vi "BMark_Highlight Object.vi"(6 "Poly Path":path, 7 "Analysis App Ref":refnum<vi>, 8 "error in (no error)":errorcluster, 10 "Run Prog?":bool, 11 "GObj Refnum":refnum<vi>) -> (0 "error out":errorcluster)   [LabVIEW 2016]
uses:
  <resource>/dialog/BookmarkManager/managers/Default/globals/BMark_User Visible Strings.vi
panel:
  # "Copied from VIAnRes Highlight Object.vi"
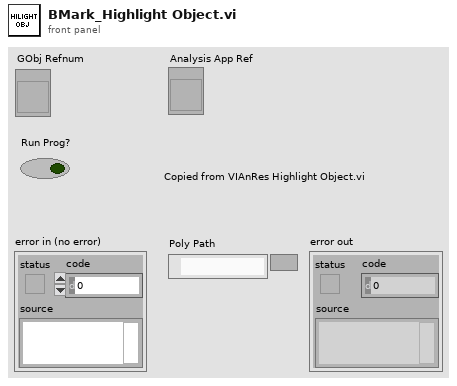
[diagram p1: front panel]
types:
  T1 = enum32{"invalid VI type", "Standard VI", "Control VI", "Global VI", "Polymorphic VI", "Configuration VI"}
  T2 = enum32{"Bad", "Idle", "Run top level", "Running"}
  T3 = enum32{"invalid VI type", "Standard VI", "Control VI", "Global VI", "Polymorphic VI", "Configuration VI", "SubSystem", "Facade VI", "Method VI", "Statechart Diagram VI"}
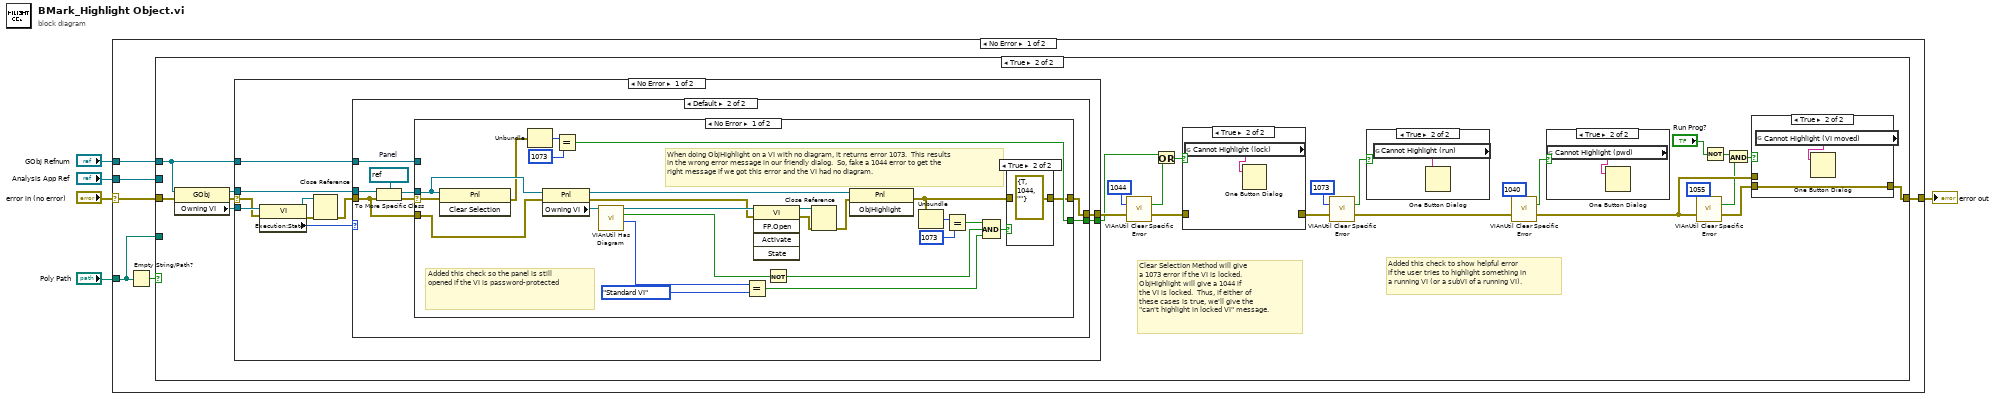
[diagram p0: block diagram]
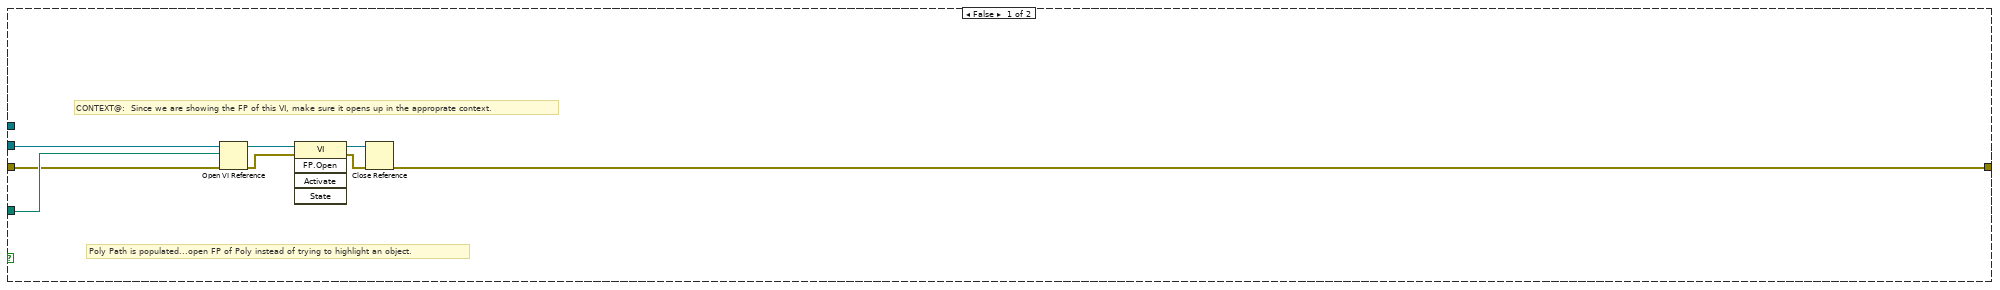
[diagram p2: hidden frame]
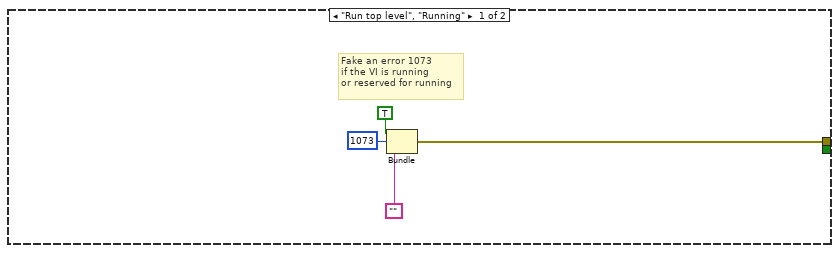
[diagram p3: hidden frame]
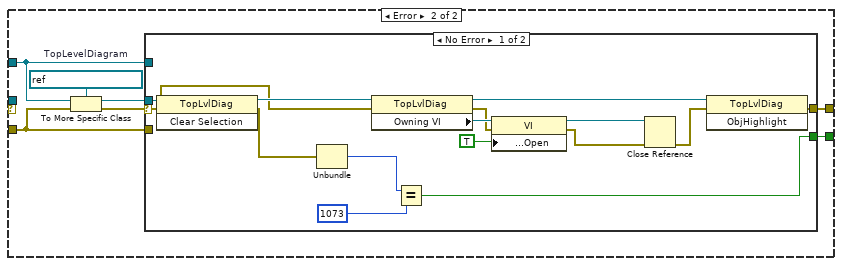
[diagram p5: hidden frame]
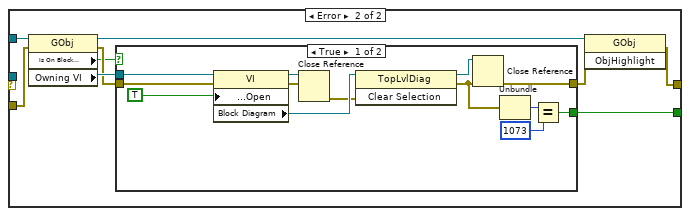
[diagram p6: hidden frame]
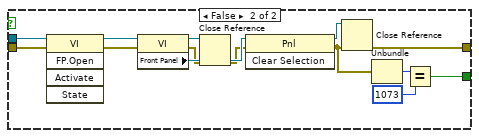
[diagram p7: hidden frame]
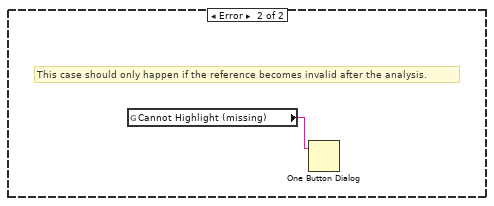
[diagram p8: hidden frame]
diagram:
  n1 = case shown="No Error" "error in (no error)" {
    selector: "error in (no error)" -> [w9 w160]
    tunnel: "GObj Refnum" -> [w10 _]
    tunnel: [w11 w160] -> w3
    tunnel: "Poly Path" -> [w7 _]
    tunnel: "Analysis App Ref" -> [w6 _]
    frame No Error {
      n2 = Empty String/Path?(string/path=w7) -> (empty?=w8:bool)
      n3 = case shown="True" w8 {
        tunnel: [w17 w32] -> w11
        tunnel: w10 -> [_ w29]
        tunnel: w9 -> [w18 w30]
        tunnel: w7 -> [w19 _]
        tunnel: w6 -> [w16 _]
        frame False {
          # "CONTEXT@:  Since we are showing the FP of this VI, make sure it opens up in the approprate context."
          # "Poly Path is populated...open FP of Poly instead of trying to highlight an object."
          n4 = Open VI Reference(application reference (local)=w16, vi path=w19, error in (no error)=w18) -> (vi reference=w15:refnum<vi>, error out=w14:errorcluster)  [unwired: 3 in]
          n5 = invoke class="VI" method="FP.Open"(reference=w15, error in=w14) -> (reference out=w13:refnum<vi>, error out=w12:errorcluster)  [unwired: 3 in, 3 out]
          n6 = Close Reference(reference=w13, error in (no error)=w12) -> (error out=w17:errorcluster)
        }
        frame True {
          # "Clear Selection Method will give\na 1073 error if the VI is locked. \nObjHighlight will give a 1044 if\nthe VI is locked.  Thus, if either of\nthese cases is true, we'll give the\n\"can't highlight in locked VI\" message."
          # "Added this check to show helpful error\nif the user tries to highlight something in\na running VI (or a subVI of a running VI)."
          n7 = property class="GObj"(reference=w29, error in=w30) -> (reference out=w28:refnum<vi>, error out=w25:errorcluster, "Owning VI"=w31:refnum<vi>)
          n8 = case shown="No Error" w25 {
            selector: w25 -> [w46 _]
            tunnel: w31 -> [w50 _]
            tunnel: w29 -> [w49 _]
            tunnel: w28 -> [w48 _]
            tunnel: [w47 _] -> w26
            tunnel: [w45 _] -> w20
            frame No Error {
              n9 = property class="VI"(reference=w50, error in=w46) -> (reference out=w52:refnum<vi>, error out=w53:errorcluster, "Execution:State"=w54:T2)
              n10 = Close Reference(reference=w52, error in (no error)=w53) -> (error out=w51:errorcluster)
              n11 = case shown="Default" w54 {
                tunnel: w49 -> [_ w63]
                tunnel: w48 -> [_ w62]
                tunnel: [w58 w61] -> w47
                tunnel: w51 -> [_ w60]
                tunnel: [_ w59] -> w45
                frame "Run top level", "Running" {
                  # "Fake an error 1073\nif the VI is running\nor reserved for running"
                  n12 = Bundle(TRUE, "Error of Interest"=1073, "") -> (w58:cluster{bool, "Error of Interest":i32, string})  [unwired: 1 out]
                }
                frame Default {
                  w66 = refnum<vi> refnum  # Panel
                  n13 = To More Specific Class(target class=w66, reference=w62, error in=w60) -> (specific class reference=w64:refnum<vi>, error out=w65:errorcluster)
                  n14 = case shown="No Error" w65 {
                    selector: w65 -> [w90 _]
                    tunnel: w64 -> [w88 _]
                    tunnel: w63 -> [_ w98]
                    tunnel: [w72 w97] -> w61
                    tunnel: w60 -> [w83 w96]
                    tunnel: [w84 w95] -> w59
                    frame No Error {
                      # "When doing ObjHighlight on a VI with no diagram, it returns error 1073.  This results in the wrong error message in our friendly dialog.  So, fake a 1044 error to get the right message if we got this error and the VI had no diagram."
                      # "Added this check so the panel is still\nopened if the VI is password-protected"
                      n15 = invoke class="Pnl" method="Clear Selection"(reference=w88, error in=w90) -> (error out=w85:errorcluster)  [unwired: 1 in, 2 out]
                      n16 = Unbundle(w85) -> ("code"=w87:i32)  [unwired: 2 out]
                      n17 = property class="Pnl"(reference=w88, error in=w83) -> (reference out=w91:refnum<vi>, error out=w67:errorcluster, "Owning VI"=w82:refnum<vi>)
                      n18 = Equal?(x=w87, y=1073) -> (x = y?=w84:bool)
                      n19 = call <vilib>:"VIAnUtil Has Diagram.vi"("VI Ref"=w82) -> ("VI Type"=w81:T3, "Has Diag?"=w76:bool, "dup VI Ref"=w68:refnum<vi>)  [unwired: 2 in, 6 out]
                      n20 = Equal?(x=w81, y=T1."Standard VI") -> (x = y?=w75:bool)
                      n21 = invoke class="VI" method="FP.Open"(reference=w68, error in=w67) -> (reference out=w70:refnum<vi>, error out=w69:errorcluster)  [unwired: 3 in, 3 out]
                      n22 = Not(x=w76) -> (.not. x?=w71:bool)
                      n23 = Close Reference(reference=w70, error in (no error)=w69) -> (error out=w89:errorcluster)
                      n24 = invoke class="Pnl" method="ObjHighlight"(reference=w91, error in=w89) -> (error out=w73:errorcluster)  [unwired: 1 in, 2 out]
                      n25 = Unbundle(w73) -> ("code"=w79:i32)  [unwired: 2 out]
                      n26 = Equal?(x=w79, y=1073) -> (x = y?=w77:bool)
                      n27 = Compound Arithmetic op=AND(w77, w71, w75) -> (w74:bool)
                      n28 = case shown="True" w74 {
                        tunnel: w73 -> [w92 _]
                        tunnel: [w92 errorcluster {"status"=TRUE, "code"=1044, "source"=""} ("error out")] -> w72
                        frame False {
                        }
                        frame True {
                        }
                      }
                    }
                    frame Error {
                      w100 = refnum<vi> refnum  # TopLevelDiagram
                      n29 = To More Specific Class(target class=w100, reference=w98, error in=w96) -> (specific class reference=w94:refnum<vi>, error out=w99:errorcluster)
                      n30 = case shown="No Error" w99 {
                        selector: w99 -> [w101 _]
                        tunnel: w98 -> [_ w124]
                        tunnel: w94 -> [w110 _]
                        tunnel: [w111 w117] -> w97
                        tunnel: w96 -> [_ w123]
                        tunnel: [w103 w116] -> w95
                        frame No Error {
                          n31 = invoke class="TopLvlDiag" method="Clear Selection"(reference=w110, error in=w101) -> (reference out=w109:refnum<vi>, error out=w102:errorcluster)  [unwired: 1 in, 1 out]
                          n32 = Unbundle(w102) -> ("code"=w105:i32)  [unwired: 2 out]
                          n33 = property class="TopLvlDiag"(reference=w109, error in=w101) -> (reference out=w112:refnum<vi>, error out=w114:errorcluster, "Owning VI"=w115:refnum<vi>)
                          n34 = Equal?(x=w105, y=1073) -> (x = y?=w103:bool)
                          n35 = property class="VI"(reference=w115, error in=w114, "Block Diagram Window:Open"=TRUE ("Front Panel Window:Open")) -> (reference out=w108:refnum<vi>, error out=w107:errorcluster)
                          n36 = Close Reference(reference=w108, error in (no error)=w107) -> (error out=w106:errorcluster)
                          n37 = invoke class="TopLvlDiag" method="ObjHighlight"(reference=w112, error in=w106) -> (error out=w111:errorcluster)  [unwired: 1 in, 2 out]
                        }
                        frame Error {
                          n38 = property class="GObj"(reference=w124, error in=w123) -> (reference out=w122:refnum<vi>, error out=w120:errorcluster, "Is On Block Diagram?"=w119:bool, "Owning VI"=w121:refnum<vi>)
                          n39 = case shown="True" w119 {
                            tunnel: w121 -> [w137 w141]
                            tunnel: w120 -> [w136 w139]
                            tunnel: [w129 w146] -> w118
                            tunnel: [w125 w143] -> w116
                            frame True {
                              n40 = property class="VI"(reference=w137, error in=w136, "Block Diagram Window:Open"=TRUE) -> (reference out=w133:refnum<vi>, error out=w132:errorcluster, "Block Diagram"=w135:refnum<vi>)
                              n41 = Close Reference(reference=w133, error in (no error)=w132) -> (error out=w131:errorcluster)
                              n42 = invoke class="TopLvlDiag" method="Clear Selection"(reference=w135, error in=w131) -> (reference out=w130:refnum<vi>, error out=w126:errorcluster)  [unwired: 1 in, 1 out]
                              n43 = Close Reference(reference=w130, error in (no error)=w126) -> (error out=w129:errorcluster)
                              n44 = Unbundle(w126) -> ("code"=w128:i32)  [unwired: 2 out]
                              n45 = Equal?(x=w128, y=1073) -> (x = y?=w125:bool)
                            }
                            frame False {
                              n46 = invoke class="VI" method="FP.Open"(reference=w141, error in=w139) -> (reference out=w140:refnum<vi>, error out=w138:errorcluster)  [unwired: 3 in, 3 out]
                              n47 = property class="VI"(reference=w140, error in=w138) -> (reference out=w150:refnum<vi>, error out=w149:errorcluster, "Front Panel"=w151:refnum<vi>)
                              n48 = Close Reference(reference=w150, error in (no error)=w149) -> (error out=w148:errorcluster)
                              n49 = invoke class="Pnl" method="Clear Selection"(reference=w151, error in=w148) -> (reference out=w147:refnum<vi>, error out=w142:errorcluster)  [unwired: 1 in, 1 out]
                              n50 = Close Reference(reference=w147, error in (no error)=w142) -> (error out=w146:errorcluster)
                              n51 = Unbundle(w142) -> ("code"=w145:i32)  [unwired: 2 out]
                              n52 = Equal?(x=w145, y=1073) -> (x = y?=w143:bool)
                            }
                          }
                          n53 = invoke class="GObj" method="ObjHighlight"(reference=w122, error in=w118) -> (error out=w117:errorcluster)  [unwired: 1 in, 2 out]
                        }
                      }
                    }
                  }
                }
              }
            }
            frame Error {
              # "This case should only happen if the reference becomes invalid after the analysis."
              n54 = global read "BMark_User Visible Strings.vi" "Cannot Highlight (missing)"() -> (w152:string)
              n55 = One Button Dialog(message=w152) -> ()  [unwired: 2 out]
            }
          }
          n56 = call <vilib>:"VIAnUtil Clear Specific Error.vi"("Error of Interest"=1044, "error in (current)"=w26) -> ("Specific Error?"=w21:bool, "error out"=w24:errorcluster)  [unwired: 1 in, 11 out]
          n57 = Or(x=w20, y=w21) -> (x .or. y?=w22:bool)
          n58 = case shown="True" w22 {
            tunnel: w24 -> [w153 _]
            tunnel: [w153 _] -> w23
            frame False {
            }
            frame True {
              n59 = global read "BMark_User Visible Strings.vi" "Cannot Highlight (lock)"() -> (w154:string)
              n60 = One Button Dialog(message=w154) -> ()  [unwired: 2 out]
            }
          }
          n61 = call <vilib>:"VIAnUtil Clear Specific Error.vi"("Error of Interest"=1073, "error in (current)"=w23) -> ("Specific Error?"=w34:bool, "error out"=w35:errorcluster)  [unwired: 1 in, 11 out]
          n62 = case shown="True" w34 {
            frame False {
            }
            frame True {
              n63 = global read "BMark_User Visible Strings.vi" "Cannot Highlight (run)"() -> (w159:string)
              n64 = One Button Dialog(message=w159) -> ()  [unwired: 2 out]
            }
          }
          n65 = call <vilib>:"VIAnUtil Clear Specific Error.vi"("Error of Interest"=1040, "error in (current)"=w35) -> ("Specific Error?"=w37:bool, "error out"=w43:errorcluster)  [unwired: 1 in, 11 out]
          n66 = case shown="True" w37 {
            frame False {
            }
            frame True {
              n67 = global read "BMark_User Visible Strings.vi" "Cannot Highlight (pwd)"() -> (w158:string)
              n68 = One Button Dialog(message=w158) -> ()  [unwired: 2 out]
            }
          }
          n69 = call <vilib>:"VIAnUtil Clear Specific Error.vi"("Error of Interest"=1055, "error in (current)"=w43) -> ("Specific Error?"=w40:bool, "error out"=w42:errorcluster)  [unwired: 1 in, 11 out]
          n70 = Not(x="Run Prog?") -> (.not. x?=w44:bool)
          n71 = And(x=w44, y=w40) -> (x .and. y?=w41:bool)
          n72 = case shown="True" w41 {
            tunnel: w42 -> [_ w157]
            tunnel: w43 -> [w155 _]
            tunnel: [w155 w157] -> w32
            frame False {
            }
            frame True {
              n73 = global read "BMark_User Visible Strings.vi" "Cannot Highlight (VI moved)"() -> (w156:string)
              n74 = One Button Dialog(message=w156) -> ()  [unwired: 2 out]
            }
          }
        }
      }
    }
    frame Error {
    }
  }
  "error out" <- w3
